vi "4-20mA Module (Main).vi"(7 "Name of Parent Panel":string="Main.vi", 9 "New Center Coords":T1={"Horizontal"=470, "Vertical"=200}, 10 "Config":variant, 11 "Main UI Message Queue":refnum<queue>) -> ()   [LabVIEW 2018, in "4-20mA Module.lvlib"]
doc: "This Continuous Measurement sample project is based on the Queued Message Handler template.\n\nThe Event Handling Loop generates messages based on user interface actions.\n\nThe Message Handling Loop processes messages generated by the Event Handling Loop, or by other messages. There are also Acquisition and Logging message handling loop subVIs, and a chart updating loop."
uses:
  4-20mA Module.lvlib
  support/Message Queue/Message Cluster.ctl
  <vilib>/Utility/miscctls.llb/LVPoint32TypeDef.ctl
  controls/UI Data.ctl
  controls/UI State.ctl
  Controls/4-20mA Module State Cluster.ctl
  Controls/4-20mA Module Config Cluster.ctl
  Controls/4-20mA Module Settings Cluster.ctl
  Pressure Transmitter/Pressure Transmitter Device Settings.ctl
  Pressure Reg Module/Pressure Regulator Device Settings.ctl
  Measure Instrument/State Enum.ctl
  Sequencing/Squence Update Cluster.ctl
  Controls/4-20mA Display Cluster.ctl
  Tag VIs/Tag FGV Operation Enum.ctl
  support/Message Queue/Enqueue Message (Single).vi
  support/User Event - Stop/User Event - Stop.lvlib
  support/Support Library.lvlib
  support/Message Queue/Message Queue.lvlib
  Measure Instrument/4-20mA Module Engine.lvlib
  Sequencing/Sequencing Library.lvlib
  Pressure Transmitter/Pressure Transmitter Library.lvlib
  Pressure Reg Module/Pressure Regulator Library.lvlib
  Shared Variables/Dynamic Shared Variables.lvlib
  Measure Instrument/Feed Module Engine.lvlib
  support/Command Log VIs/Command Logging.lvlib
  Settings Dialog.vi
  Report Generation/Report Generation.lvlib
panel:
  in  "Settings Dialog Button":bool
  out "User name":string
  out "Original Width 3":u32
  out "Original Width 2":u32
  out "Display Cluster":cluster{"Input":dbl, "Output":dbl} {"Output" format="%.2f"; "Input" format="%.2f"}
  out "Image Status":u16(ring)=2
  out "H/W":dbl
  out "Original Height":u32
  out "Original Width":u32
  out "Input Channel":string
  out "Log File path":path
  out "Status":string
  in  "Exit":bool
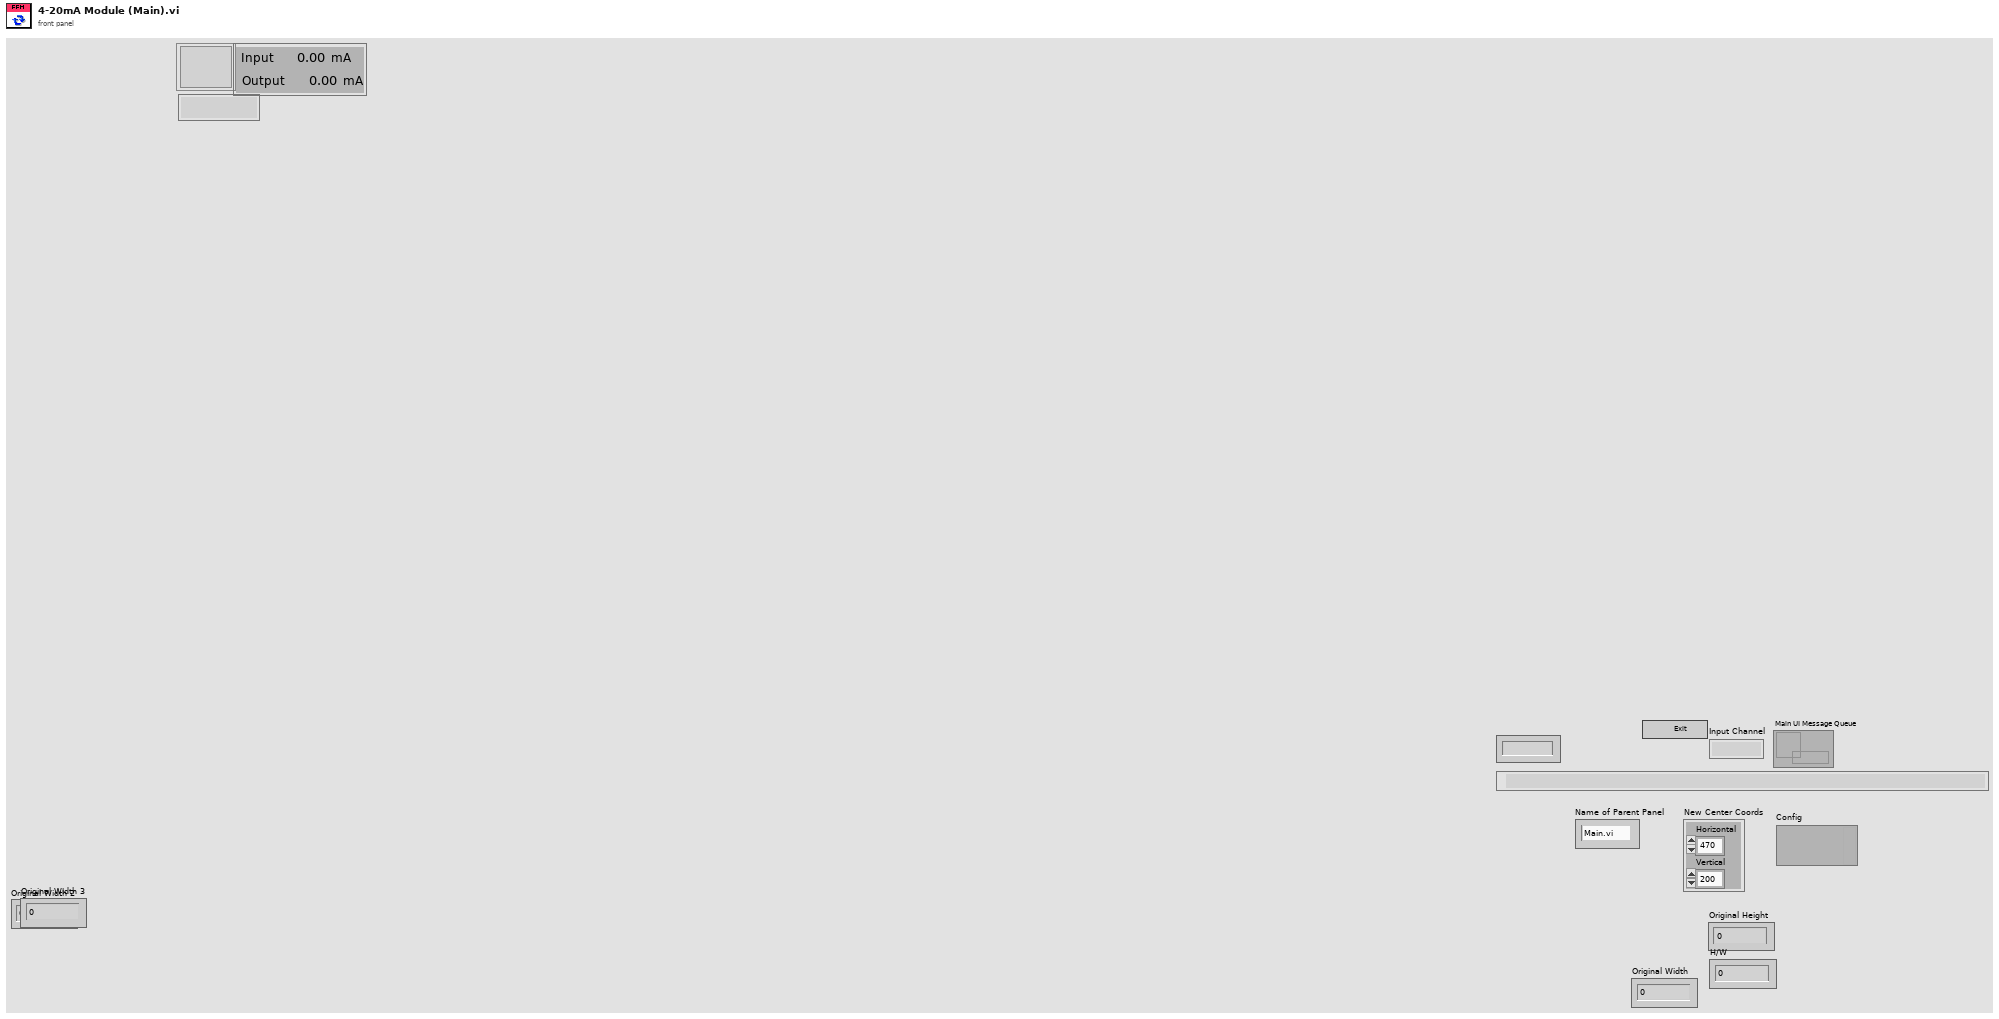
[diagram p1: front panel]
types:
  T1 = typedef "LVPoint32TypeDef.ctl" = cluster{"Horizontal":i32, "Vertical":i32}
  T2 = enum32{"Invalid", "Default", "Floating", "Floating/Auto-Hide", "Modal"}
  T3 = typedef "4-20mA Module.lvlib/4-20mA Module Config Cluster.ctl" = cluster{"GUID":string, "Drop Coords":T1, "Process Name":string, "User name":string, "Queue Name":string, "Settings":T4, "Settings Load Count":i32}
  T4 = typedef "4-20mA Module.lvlib/4-20mA Module Settings Cluster.ctl" = cluster{"Cycle Period":dbl, "PID 2 Parameters":cluster{"Input Device":enum16{"Default", "4-20mA"}, "Output Device":enum16{"Default", "Equilibar Pressure Reg", "Flow Regulator"}, "Setpoint":dbl, "PID gains":cluster{"proportional gain (Kc)":dbl, "integral time (Ti, min)":dbl, "derivative time (Td, min)":dbl}, "output range":cluster{"output low":dbl, "output high":dbl}}, "Manual Entry":dbl, "Auto?":bool, "4-20mA Input Settings":T5, "4-20mA Out Settings":T6, "Input Channel Tag Name ":string}
  T5 = typedef "Pressure Transmitter Library.lvlib/Pressure Transmitter Device Settings.ctl" = cluster{"Input Channel ":u16}
  T6 = typedef "Pressure Regulator Library.lvlib/Pressure Regulator Device Settings.ctl" = cluster{"Output DAQ Task":refnum<k21>}
  T7 = typedef "UI State.ctl" = enum16{"Idle", "Acquiring and Logging", "Waiting for Exit", "Waiting for Exit (Acq Stopped)", "Waiting for Exit (Log Stopped)", "Waiting for Stop", "Waiting for Stop (Acq Stopped)", "Waiting for Stop (Log Stopped)"}
  T8 = typedef "UI Data.ctl" = cluster{"Start Ref":refnum<vi>, "Trigger Ref":refnum<vi>, "Stop Ref":refnum<vi>, "Settings Ref":refnum<vi>, "Status Ref":refnum<vi>, "Exit Ref":refnum<vi>, "Data Ref":refnum<vi>}
  T9 = typedef "4-20mA Module.lvlib/4-20mA Module State Cluster.ctl" = cluster{"PRM Config":T3, "State":T10, "Start Time":timestamp, "Current Time":timestamp, "First Iteration":bool, "Data":cluster{"4-20mA Input":dbl, "PID 2 Process Variable":dbl, "PID 2 Output":dbl, "4-20mA Output":dbl}}
  T10 = typedef "Feed Module.lvlib/Feed Module Engine.lvlib/State Enum.ctl" = enum16{"Measuring", "Idle", "Paused"}
  T11 = typedef "LVPointTypeDef.ctl" = cluster{"Horizontal":i16, "Vertical":i16}
  T12 = typedef "4-20mA Module.lvlib/4-20mA Message Queues.ctl" = cluster{"UI":refnum<queue>, "Engine":refnum<queue>, "PR Display":refnum<queue>, "Setting Display":refnum<queue>}
  T13 = typedef "4-20mA Module.lvlib/4-20mA Display Cluster.ctl" = cluster{"Input 4-20":dbl, "Output 4-20":dbl, "Cycle Period":dbl, "Status":enum16{"Off", "On", "Not Initialized"}}
  T14 = typedef "Tag FGV Operation Enum.ctl" = enum16{"Init", "Set Notification Queue", "Create Tag", "Commit", "Write Tag (Numeric)", "Write Tag (Boolean)", "Read All Tags", "Read One Tag", "Delete Tag Category", "Set Alarm Parameters (Numeric)", "Set Alarm Parameters (Boolean)", "Enable All Alarms", "Disable All Alarms", "Delete All Tags", "Read Alarms", "Ack Alarm", "Read Alarm Parameters (Numeric)", "Read Alarm Parameters (Boolean)"}
  T15 = typedef "LVRectTypeDef.ctl" = cluster{"Left":i16, "Top":i16, "Right":i16, "Bottom":i16}
  T16 = cluster{"Shift":bool, "Ctrl":bool, "Alt":bool, "Cmd":bool, "Opt":bool}
  T17 = typedef "Sequencing Library.lvlib/Squence Update Cluster.ctl" = cluster{"Auto?":bool, "Manual Entry":dbl, "Setpoint":dbl}
  T18 = enum8{"Enabled", "Disabled", "Disabled and Grayed Out"}
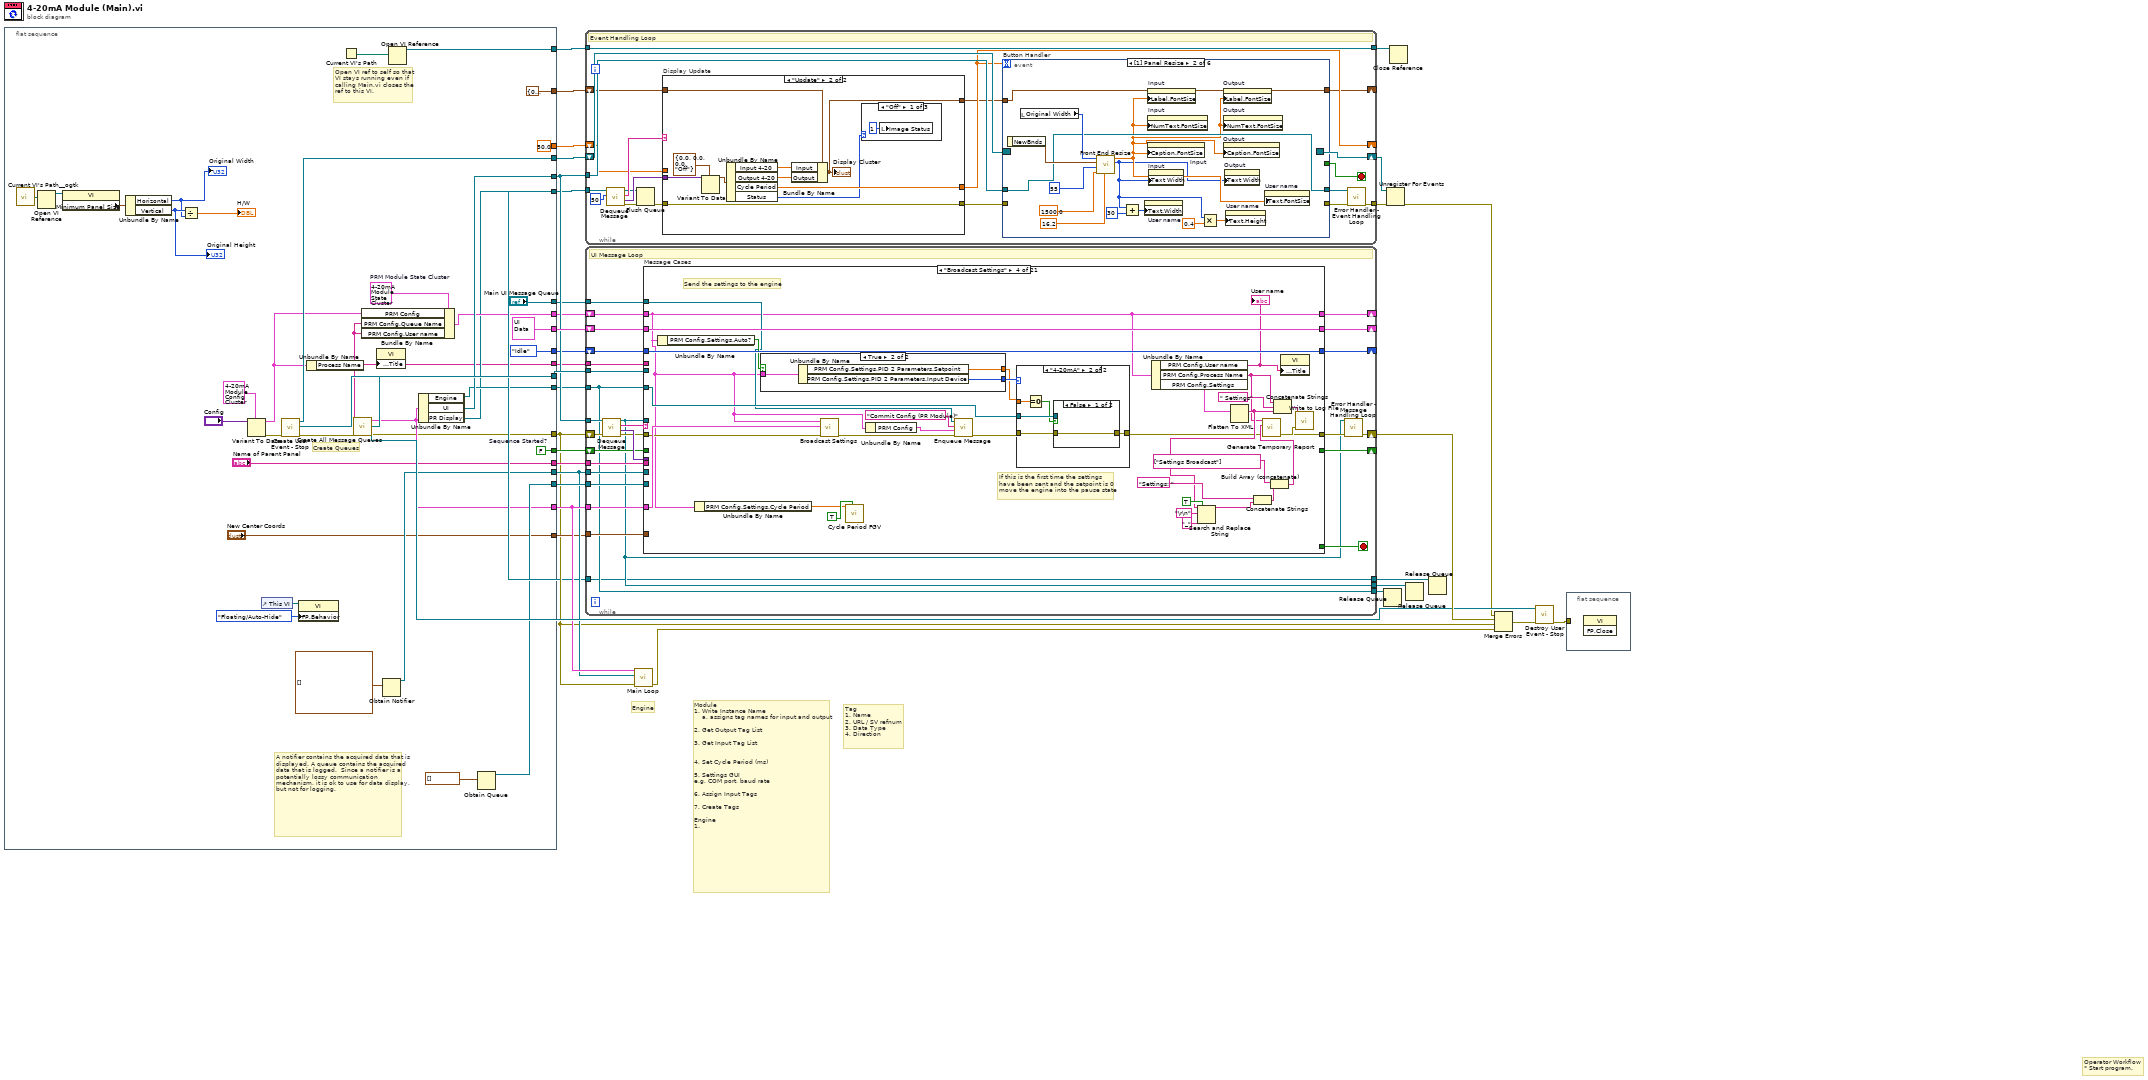
[diagram p0: block diagram]
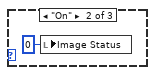
[diagram p3: hidden frame]
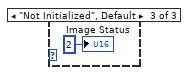
[diagram p4: hidden frame]
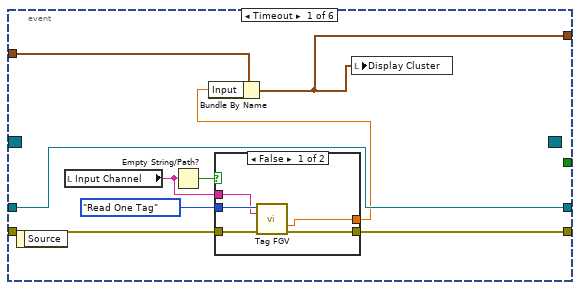
[diagram p5: hidden frame]
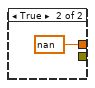
[diagram p6: hidden frame]
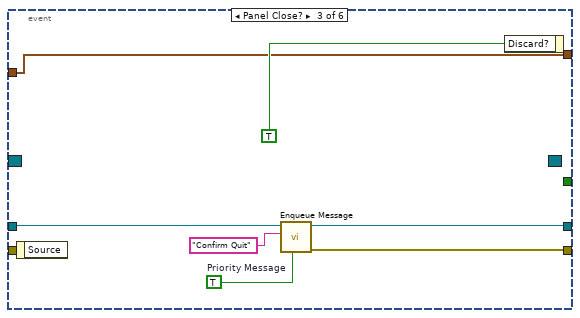
[diagram p7: hidden frame]
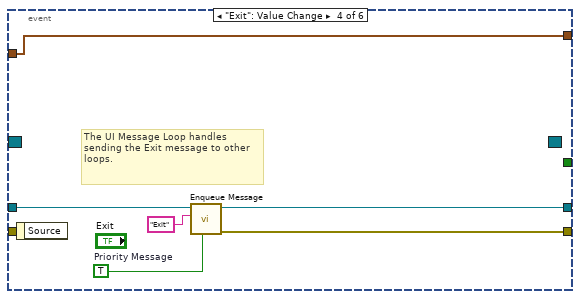
[diagram p8: hidden frame]
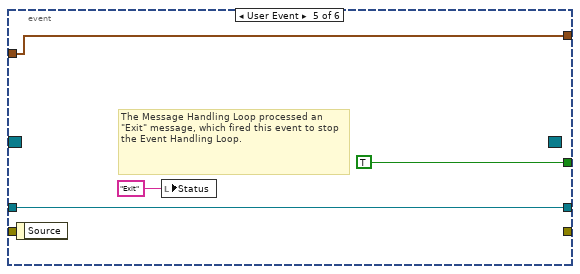
[diagram p9: hidden frame]
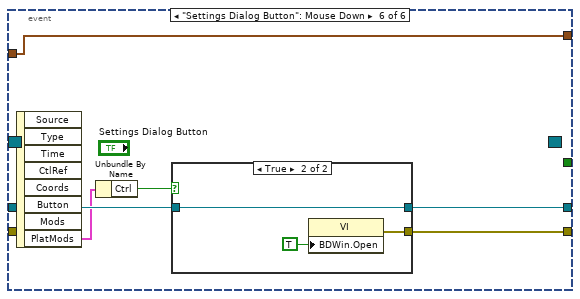
[diagram p10: hidden frame]
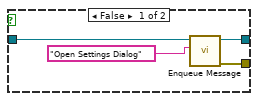
[diagram p11: hidden frame]
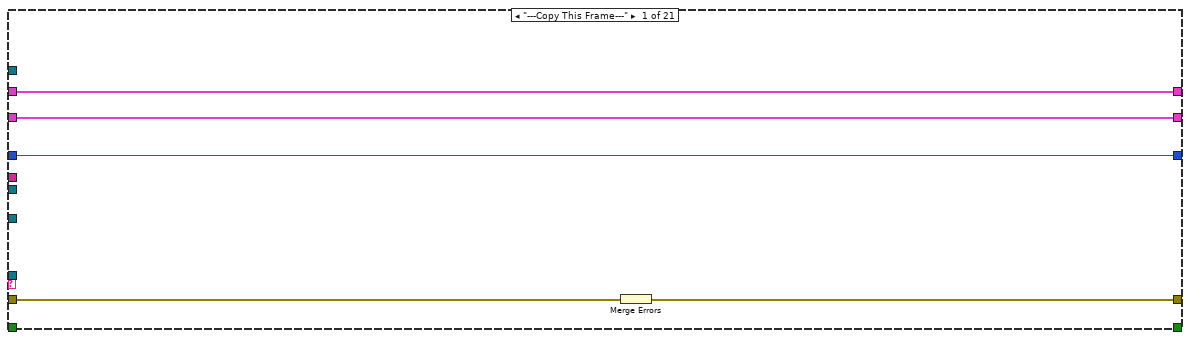
[diagram p12: hidden frame]
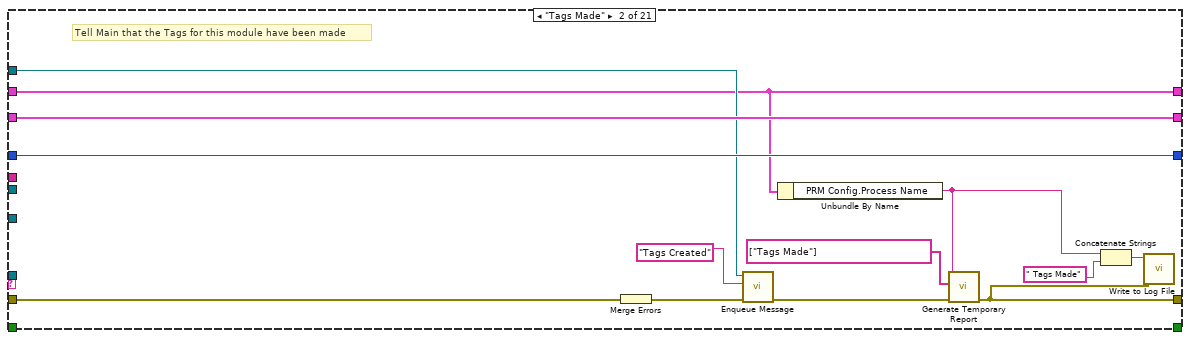
[diagram p13: hidden frame]
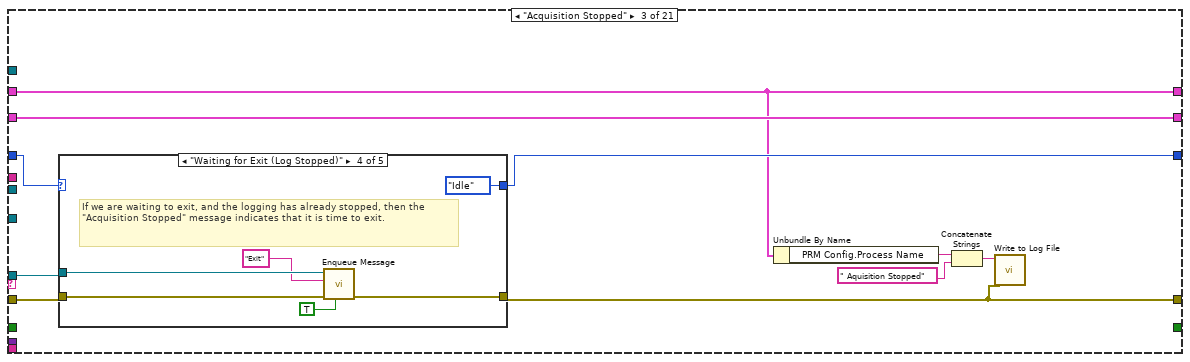
[diagram p14: hidden frame]
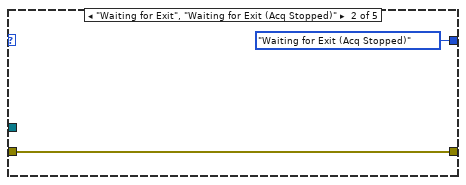
[diagram p16: hidden frame]
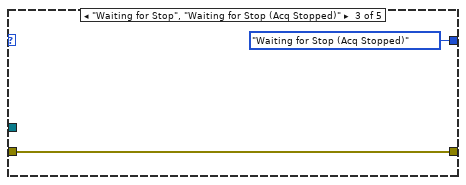
[diagram p17: hidden frame]
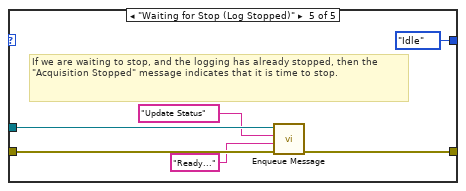
[diagram p18: hidden frame]
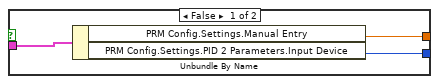
[diagram p19: hidden frame]
diagram:
  # "Engine"
  # "Operator Workflow\n* Start program."
  # "Module \n1. Write Instance Name\n    a. assigns tag names for input and output\n\n2. Get Output Tag List\n\n3. Get Input Tag List\n\n\n4. Set Cycle Period (ms)\n\n5. Settings GUI\ne.g. COM port, baud rate\n\n6. Assign Input Tags\n\n7. Create Tags\n\nEngine\n1."
  # "Tag\n1. Name\n2. URL / SV refnum\n3. Data Type\n4. Direction"
  n1 = flat-sequence {
    tunnel: [w68] -> w28
    tunnel: [w67] -> w27
    tunnel: [T8 {"Start Ref"=refnum, "Trigger Ref"=refnum, "Stop Ref"=refnum, "Settings Ref"=refnum, "Status Ref"=refnum, "Exit Ref"=refnum, "Data Ref"=refnum} ("Measurement UI Controls")] -> w24
    tunnel: [w64] -> w23
    tunnel: [UI_State."Idle" ("UI State")] -> w22
    tunnel: [w60] -> w21
    tunnel: [w59] -> w20
    tunnel: [w58] -> w18
    tunnel: [w57] -> w17
    tunnel: [w56] -> w15
    tunnel: ["Main UI Message Queue"] -> w14
    tunnel: ["Name of Parent Panel"] -> w13
    tunnel: ["New Center Coords"] -> w12
    tunnel: [w48] -> w10
    tunnel: [w47] -> w9
    tunnel: [w44] -> w8
    tunnel: [50.0 ("Cycle Period")] -> w7
    tunnel: [w42] -> w4
    tunnel: [w39] -> w2
    tunnel: [cluster{"Input":dbl, "Output":dbl} {"Input"=0.0, "Output"=0.0} ("Display Cluster 2")] -> w1
    frame #0 {
      w48 = FALSE  # Sequence Started?
      w51 = T9 {"PRM Config"={"GUID"="", "Drop Coords"={"Horizontal"=0, "Vertical"=0}, "Process Name"="", "User name"="", "Queue Name"="", "Settings"={"Cycle Period"=500.0, "PID 2 Parameters"={"Input Device"=enum."Default", "Output Device"=enum."Default", "Setpoint"=0.0, "PID gains"={"proportional gain (Kc)"=1.0, "integral time (Ti, min)"=0.01, "derivative time (Td, min)"=0.0}, "output range"={"output low"=0.0, "output high"=100.0}}, "Manual Entry"=0.0, "Auto?"=TRUE, "4-20mA Input Settings"={"Input Channel "=0}, "4-20mA Out Settings"={"Output DAQ Task"=""}, "Input Channel Tag Name "=""}, "Settings Load Count"=0}, "State"=enum."Idle", "Start Time"=timestamp(0 s since 1904-01-01), "Current Time"=timestamp(0 s since 1904-01-01), "First Iteration"=FALSE, "Data"={"4-20mA Input"=0.0, "PID 2 Process Variable"=0.0, "PID 2 Output"=0.0, "4-20mA Output"=0.0}}  # PRM Module State Cluster
      # "Create Queues"
      # "Open VI ref to self so that\nVI stays running even if\ncalling Main.vi closes the\nref to this VI."
      # "A notifier contains the acquired data that is displayed. A queue contains the acquired data that is logged.  Since a notifier is a potentially lossy communication mechanism, it is ok to use for data display, but not for logging."
      n2 = call <userlib>:"Current VI's Path__ogtk.vi"() -> ("Current VI's Path (+ Relative)"=w33:path)  [unwired: 1 in]
      n3 = Open VI Reference(vi path=w33) -> (vi reference=w34:refnum<vi>)  [unwired: 5 in, 1 out]
      n4 = property class="VI"(reference=w34) -> ("Minimum Panel Size"=w35:T11)  [unwired: 1 in, 2 out]
      n5 = Unbundle By Name(w35) -> ("Horizontal"=w36:i16, "Vertical"=w37:i16)
      "Original Width" <- w36
      "Original Height" <- w37
      n6 = Divide(x=w37, y=w36) -> (x/y=→"H/W":dbl)
      n7 = Variant To Data(type=T3 {"GUID"="", "Drop Coords"={"Horizontal"=0, "Vertical"=0}, "Process Name"="", "User name"="", "Queue Name"="", "Settings"={"Cycle Period"=500.0, "PID 2 Parameters"={"Input Device"=enum."Default", "Output Device"=enum."Default", "Setpoint"=0.0, "PID gains"={"proportional gain (Kc)"=1.0, "integral time (Ti, min)"=0.01, "derivative time (Td, min)"=0.0}, "output range"={"output low"=0.0, "output high"=100.0}}, "Manual Entry"=0.0, "Auto?"=TRUE, "4-20mA Input Settings"={"Input Channel "=0}, "4-20mA Out Settings"={"Output DAQ Task"=""}, "Input Channel Tag Name "=""}, "Settings Load Count"=0} ("Feed Module Config"), Variant="Config") -> (data=w53:T3, error out=w54:errorcluster)  [unwired: 1 in]
      n8 = control-ref of="This VI"() -> (w41:refnum<vi>)
      n9 = call "Create User Event - Stop.vi"("error in (no error)"=w54) -> ("error out"=w66:errorcluster, "User Event - Stop"=w67:refnum<user-event>, "Stop Event Registration Refnum"=w68:refnum<event-registration>)  [unwired: 8 in]
      n10 = property class="VI"(reference=w41, "FP.Behavior"=T2."Floating/Auto-Hide" ("Front Panel Window:Behavior")) -> ()  [unwired: 1 in, 2 out]
      n11 = Unbundle By Name(w53) -> ("Process Name"=w39:string)
      n12 = Current VI's Path() -> (path=w55:path)
      n13 = call "Create All Message Queues.vi"("error in (no error)"=w66, "Process Name"=w39) -> ("error out"=w47:errorcluster, "Message Queues"=w58:T12)  [unwired: 8 in]
      n14 = Bundle By Name(cluster=w51, "PRM Config"=w53, "PRM Config.Queue Name"=w39, "PRM Config.User name"=w39) -> (w44:T9)
      n15 = property class="VI"("Front Panel.Title"=w39) -> ()  [unwired: 2 in, 2 out]
      n16 = Obtain Notifier(notification data type=waveform(dbl)[] []) -> (notifier out=w57:refnum<notifier>)  [unwired: 3 in, 2 out]
      n17 = Open VI Reference(vi path=w55) -> (vi reference=w56:refnum<vi>)  [unwired: 5 in, 1 out]
      n18 = Unbundle By Name(w58) -> ("Engine"=w60:refnum<queue>, "UI"=w64:refnum<queue>, "PR Display"=w42:refnum<queue>)
      n19 = Obtain Queue(element data type=waveform(dbl)[] []) -> (queue out=w59:refnum<queue>)  [unwired: 4 in, 2 out]
    }
  }
  n20 = while {
    tunnel: w23 -> [w83]
    tunnel: [w85] -> w30
    shift-right: [w84] -> w25
    shift-left: w28 -> [w89]
    tunnel: [w82] -> w16
    tunnel: w15 -> [w82]
    tunnel: w4 -> [w81]
    shift-right: [w78] -> _
    shift-left: w7 -> [w77]
    shift-right: [w70] -> _
    shift-left: w1 -> [w69]
    stop <- w88 stop-if-true
    # "Event Handling Loop"
    n21 = call "Dequeue Message.vi"("timeout in ms (-1)"=50, "Message Queue"=w81) -> ("error out"=w74:errorcluster, "Message Data"=w79:variant, "Message"=w80:string, "dup Message Queue"=w75:refnum<queue>)  [unwired: 6 in]
    n22 = Flush Queue(queue=w75, error in (no error)=w74) -> (error out=w72:errorcluster)  [unwired: 2 out]
    n23 = case "Display Update" shown="\"Update\"" w80 {
      tunnel: w79 -> [_ w102]
      tunnel: [w92 w99] -> w78
      tunnel: w77 -> [w92 _]
      tunnel: [w91 w98] -> w73
      tunnel: w72 -> [w91 w98]
      tunnel: [w90 w94] -> w71
      tunnel: w69 -> [w90 w93]
      frame "False", Default {
      }
      frame "Update" {
        n24 = Variant To Data(type=T13 {"Input 4-20"=0.0, "Output 4-20"=0.0, "Cycle Period"=0.0, "Status"=enum."Off"} ("PRM Display Cluster"), Variant=w102) -> (data=w101:T13)  [unwired: 1 in, 1 out]
        n25 = Unbundle By Name(w101) -> ("Input 4-20"=w96:dbl, "Output 4-20"=w95:dbl, "Cycle Period"=w99:dbl, "Status"=w97:enum16{"Off", "On", "Not Initialized"})
        n26 = Bundle By Name(cluster=w93, "Input"=w96, "Output"=w95) -> (w94:cluster{"Input":dbl, "Output":dbl})
        "Display Cluster" <- w94
        n27 = case shown="\"Off\"" w97 {
          frame "Off" {
            n28 = local write "Image Status"(u16 1 ("Ring")) -> ()
          }
          frame "On" {
            n29 = local write "Image Status"(u16 0 ("Ring")) -> ()
          }
          frame "Not Initialized", Default {
            "Image Status" <- u16 2 ("Ring")
          }
        }
      }
    }
    n30 = event "Button Handler" shown="[1] Panel Resize" {
      selector: w89 -> [_ _ _ _ _ _]
      dyn-events: [_ _ _ _ _ _] -> w84
      timeout: w78 -> [_ _ _ _ _ _]
      tunnel: [_ _ _ _ TRUE ("Discard?") _] -> w88
      tunnel: w83 -> [w114 w127 w137 w143 w148 w154]
      tunnel: [w109 _ w135 w146 _ w156] -> w86
      tunnel: [w114 w127 w136 w142 w148 w155] -> w87
      tunnel: w73 -> [w110 _ _ _ _ _]
      tunnel: w71 -> [w107 w133 w134 w141 w147 w151]
      tunnel: [w106 w133 w134 w141 w147 w151] -> w70
      event Timeout {
        n31 = event-data() -> ()  [unwired: 1 in, 1 out]
        n32 = local read "Input Channel"() -> (w111:string)
        n33 = Empty String/Path?(string/path=w111) -> (empty?=w113:bool)
        n34 = case shown="False" w113 {
          tunnel: Tag_FGV_Operation_Enum."Read One Tag" ("Operation") -> [w119 _]
          tunnel: [w118 nan ("Tag Value")] -> w108
          tunnel: [w117 _] -> w109
          tunnel: w111 -> [w116 _]
          tunnel: w110 -> [w115 _]
          frame False {
            n35 = call "Tag FGV.vi"("Operation"=w119, "Tag Name"=w116, "error in (no error)"=w115) -> ("Tag Value"=w118:dbl, "error out"=w117:errorcluster)  [unwired: 5 in, 6 out]
          }
          frame True {
          }
        }
        n36 = Bundle By Name(cluster=w107, "Input"=w108) -> (w106:cluster{"Input":dbl, "Output":dbl})
        n37 = local write "Display Cluster"(w106) -> ()
      }
      event Panel Resize {
        n38 = event-data() -> ("NewBnds"=w132:T15)  [unwired: 1 in]
        n39 = local read "Original Width"() -> (w131:u32)
        n40 = call "Front End Resize.vi"("Starting Font"=16.2, "Area to Font Division"=1500.0, "Original Text Box Width"=55, "NewBnds"=w132, "Original Panel Width"=w131) -> ("New Text Box Width"=w122:u64, "New Font Size"=w126:dbl)  [unwired: 5 in]
        n41 = Add(x=w122, y=u64 30) -> (x+y=w124:u64)
        n42 = property on="User name" class="Str"("Text.Width"=w124) -> ()  [unwired: 2 in, 2 out]
        n43 = property on="Input" class="DigNum (strict)"("Label.FontSize"=w126) -> ()  [unwired: 2 in, 2 out]
        n44 = property on="Input" class="DigNum (strict)"("NumText.FontSize"=w126) -> ()  [unwired: 2 in, 2 out]
        n45 = property on="Input" class="DigNum (strict)"("Caption.FontSize"=w126) -> ()  [unwired: 2 in, 2 out]
        n46 = property on="Input" class="DigNum (strict)"("Text Width"=w122) -> ()  [unwired: 2 in, 2 out]
        n47 = Multiply(x=w122, y=0.4) -> (x*y=w121:dbl)
        n48 = property on="Output" class="DigNum (strict)"("Label.FontSize"=w126) -> ()  [unwired: 2 in, 2 out]
        n49 = property on="Output" class="DigNum (strict)"("NumText.FontSize"=w126) -> ()  [unwired: 2 in, 2 out]
        n50 = property on="Output" class="DigNum (strict)"("Caption.FontSize"=w126) -> ()  [unwired: 2 in, 2 out]
        n51 = property on="Output" class="DigNum (strict)"("Text Width"=w122) -> ()  [unwired: 2 in, 2 out]
        n52 = property on="User name" class="Str"("Text.Height"=w121) -> ()  [unwired: 2 in, 2 out]
        n53 = property on="User name" class="Str"("Text.FontSize"=w126) -> ()  [unwired: 2 in, 2 out]
      }
      event Panel Close? {
        w138 = TRUE  # Priority Message
        n54 = event-data() -> ()  [unwired: 1 in, 1 out]
        n55 = call-poly "Enqueue Message.vi"("Priority Message? (F)"=w138, "Message"="Confirm Quit", "Message Queue"=w137) -> ("error out"=w135:errorcluster, "dup Message Queue"=w136:refnum<queue>)  [unwired: 7 in]
        n56 = event-data("Discard?"=TRUE) -> ()  [unwired: 1 in, 1 out]
      }
      event "Exit": Value Change {
        w144 = TRUE  # Priority Message
        # "The UI Message Loop handles sending the Exit message to other loops."
        n57 = event-data() -> ()  [unwired: 1 in, 1 out]
        n58 = call-poly "Enqueue Message.vi"("Priority Message? (F)"=w144, "Message"="Exit", "Message Queue"=w143) -> ("error out"=w146:errorcluster, "dup Message Queue"=w142:refnum<queue>)  [unwired: 7 in]
      }
      event User Event {
        # "The Message Handling Loop processed an \"Exit\" message, which fired this event to stop the Event Handling Loop."
        n59 = event-data() -> ()  [unwired: 1 in, 1 out]
        n60 = local write "Status"("Exit" ("Exit String")) -> ()
      }
      event "Settings Dialog Button": Mouse Down {
        n61 = event-data() -> ("PlatMods"=w153:T16)  [unwired: 1 in, 7 out]
        n62 = Unbundle By Name(w153) -> ("Ctrl"=w152:bool)
        n63 = case shown="True" w152 {
          tunnel: [w160 w161] -> w156
          tunnel: [w159 w162] -> w155
          tunnel: w154 -> [w158 w162]
          frame False {
            n64 = call-poly "Enqueue Message.vi"("Message"="Open Settings Dialog", "Message Queue"=w158) -> ("error out"=w160:errorcluster, "dup Message Queue"=w159:refnum<queue>)  [unwired: 8 in]
          }
          frame True {
            n65 = property class="VI"("BDWin.Open"=TRUE ("Block Diagram Window:Open")) -> (error out=w161:errorcluster)  [unwired: 2 in, 1 out]
          }
        }
      }
    }
    n66 = call "Error Handler - Event Handling Loop.vi"("error in (no error)"=w86, "Message Queue"=w87) -> ("dup error in"=w85:errorcluster)  [unwired: 8 in, 1 out]
  }
  n67 = while {
    tunnel: w23 -> [w185]
    tunnel: w27 -> [w189]
    shift-right: [w180] -> w31
    shift-left: w9 -> [w188]
    shift-right: [w183] -> _
    shift-left: w24 -> [w184]
    tunnel: w17 -> [w172]
    tunnel: w20 -> [w182]
    shift-right: [w179] -> _
    shift-left: w22 -> [w174]
    tunnel: w21 -> [w166]
    tunnel: w18 -> [w171]
    tunnel: w14 -> [w175]
    tunnel: w13 -> [w178]
    tunnel: w2 -> [w177]
    tunnel: w12 -> [w176]
    shift-right: [w169] -> _
    shift-left: w10 -> [w170]
    shift-right: [w167] -> _
    shift-left: w8 -> [w168]
    tunnel: [w166] -> w6
    tunnel: [w165] -> w5
    tunnel: [w164] -> w3
    tunnel: w4 -> [w164]
    stop <- w190 stop-if-true
    # "UI Message Loop"
    n68 = call "Dequeue Message.vi"("error in (no error)"=w188, "Message Queue"=w185) -> ("error out"=w173:errorcluster, "Message Data"=w186:variant, "Message"=w187:string, "dup Message Queue"=w165:refnum<queue>)  [unwired: 6 in]
    n69 = case "Message Cases" shown="\"Broadcast Settings\"" w187 {
      selector: w187 -> [_ _ _ _ _ _ _ _ _ _ _ _ _ _ _ _ _ _ _ _ w651]
      tunnel: w165 -> [_ _ w214 _ w293 _ w351 w367 w399 w427 _ w467 w483 w499 w532 w550 _ _ w626 _ _]
      tunnel: w173 -> [w195 w208 w215 w263 w292 w319 w336 w366 w402 w430 w452 w462 _ w500 w525 w548 w576 w588 w611 w639 _]
      tunnel: [w194 w196 w210 w238 w287 w320 w325 w355 w390 w404 w452 w454 w476 w495 w531 w541 w573 w596 w604 w640 w646] -> w181
      tunnel: [_ _ _ _ _ _ _ _ _ TRUE _ _ _ _ _ _ _ _ _ _ _] -> w190
      tunnel: w186 -> [_ _ _ _ _ w322 _ _ w401 w416 _ _ w482 _ _ _ _ _ _ w638 _]
      tunnel: w189 -> [_ _ _ _ _ _ _ _ _ w429 _ _ _ _ _ _ _ _ _ _ _]
      tunnel: w184 -> [w193 w207 w218 w268 w295 w324 w348 w364 w403 w428 w451 w463 w485 w503 w533 w564 w582 w595 w623 w635 w654]
      tunnel: [w193 w207 w218 w268 w295 w324 w348 w364 w403 w428 w450 w463 w485 w503 w533 w564 w582 w595 w623 w635 w654] -> w183
      tunnel: w182 -> [_ _ _ _ _ _ _ _ _ w422 _ _ _ _ _ _ _ _ _ _ _]
      tunnel: w174 -> [w192 w206 w217 w267 w294 w318 w337 _ w394 _ _ _ w484 w502 w528 _ _ _ w612 w630 w653]
      tunnel: [w192 w206 w216 w267 w291 w318 w338 UI_State."Acquiring and Logging" ("UI State") w394 UI_State."Idle" ("UI State") UI_State."Idle" ("UI State") UI_State."Idle" ("UI State") w484 w501 w528 UI_State."Acquiring and Logging" ("UI State") UI_State."Acquiring and Logging" ("UI State") UI_State."Acquiring and Logging" ("UI State") w613 w630 w653] -> w179
      tunnel: w166 -> [_ _ _ w262 _ _ w335 _ _ w420 _ _ _ _ _ _ w580 w593 w610 _ _]
      tunnel: w178 -> [_ _ _ _ _ _ _ _ _ _ _ w461 _ _ _ _ _ _ _ _ _]
      tunnel: w177 -> [_ _ _ _ _ _ _ _ _ _ _ w458 _ _ _ _ _ _ _ _ _]
      tunnel: w176 -> [_ _ _ _ _ _ _ _ _ _ _ w460 _ _ _ _ _ _ _ _ _]
      tunnel: w175 -> [_ w204 _ w255 _ _ _ _ _ w414 _ _ _ _ _ _ _ _ _ _ _]
      tunnel: w172 -> [_ _ _ _ _ _ _ _ _ w426 _ _ _ _ _ _ _ _ _ _ _]
      tunnel: w171 -> [_ _ _ w266 _ _ _ _ _ _ _ _ _ _ w526 _ _ _ _ _ _]
      tunnel: w168 -> [w191 w200 w209 w250 w286 w317 w329 w354 w389 w411 w443 w453 w475 w494 w529 w543 w578 w590 w603 w629 w652]
      tunnel: w170 -> [_ _ _ _ _ _ _ w363 _ _ _ _ _ _ _ _ _ _ _ _ _]
      tunnel: [_ _ _ _ _ _ _ w360 _ _ _ _ _ _ _ _ _ _ _ _ _] -> w169
      tunnel: [w191 w200 w209 w250 w286 w317 w329 w354 w389 w411 w443 w453 w474 w494 w523 w543 w578 w590 w603 w629 w652] -> w167
      frame "---Copy This Frame---" {
        # "Duplicate this frame when creating new messages.  Change this comment in the duplicated frame to describe this message."
        n70 = Merge Errors(w195) -> (w194:errorcluster)
      }
      frame "Tags Made" {
        # "Tell Main that the Tags for this module have been made"
        # "Duplicate this frame when creating new messages.  Change this comment in the duplicated frame to describe this message."
        n71 = Merge Errors(w208) -> (w203:errorcluster)
        n72 = call-poly "Enqueue Message.vi"("error in (no error)"=w203, "Message"="Tags Created", "Message Queue"=w204) -> ("error out"=w197:errorcluster)  [unwired: 7 in, 1 out]
        n73 = Unbundle By Name(w200) -> ("PRM Config.Process Name"=w198:string)
        n74 = call "Generate Temporary Report.vi"("error in (no error)"=w197, "Line of Events"=string[] ["Tags Made"], "Module Name"=w198) -> ("error out"=w196:errorcluster)  [unwired: 8 in]
        n75 = Concatenate Strings(w198, " Tags Made" ("text")) -> (w201:string)
        n76 = call "Write to Log File.vi"("error in"=w196, "text"=w201) -> ()  [unwired: 9 in, 1 out]
      }
      frame "Acquisition Stopped" {
        # "Logic for determining what action to take when the acquisition has stopped."
        n77 = case shown="\"Waiting for Exit (Log Stopped)\"" w217 {
          selector: w217 -> [w220 _ _ _ _]
          tunnel: [w220 UI_State."Waiting for Exit (Acq Stopped)" ("UI State") UI_State."Waiting for Stop (Acq Stopped)" ("UI State") UI_State."Idle" ("UI State") UI_State."Idle" ("UI State")] -> w216
          tunnel: w215 -> [w219 w221 w223 w229 w235]
          tunnel: [w219 w221 w223 w228 w234] -> w210
          tunnel: w214 -> [_ _ _ w227 w233]
          frame Default {
          }
          frame "Waiting for Exit", "Waiting for Exit (Acq Stopped)" {
          }
          frame "Waiting for Stop", "Waiting for Stop (Acq Stopped)" {
          }
          frame "Waiting for Exit (Log Stopped)" {
            # "If we are waiting to exit, and the logging has already stopped, then the \"Acquisition Stopped\" message indicates that it is time to exit."
            n78 = call-poly "Enqueue Message.vi"("Priority Message? (F)"=TRUE, "error in (no error)"=w229, "Message"="Exit", "Message Queue"=w227) -> ("error out"=w228:errorcluster)  [unwired: 6 in, 1 out]
          }
          frame "Waiting for Stop (Log Stopped)" {
            # "If we are waiting to stop, and the logging has already stopped, then the \"Acquisition Stopped\" message indicates that it is time to stop."
            n79 = call-poly "Enqueue Message.vi"("error in (no error)"=w235, "Message Data"="Ready..." ("Message"), "Message"="Update Status", "Message Queue"=w233) -> ("error out"=w234:errorcluster)  [unwired: 6 in, 1 out]
          }
        }
        n80 = Unbundle By Name(w209) -> ("PRM Config.Process Name"=w213:string)
        n81 = Concatenate Strings(w213, " Aquisition Stopped" ("text")) -> (w211:string)
        n82 = call "Write to Log File.vi"("error in"=w210, "text"=w211) -> ()  [unwired: 9 in, 1 out]
      }
      frame "Broadcast Settings" {
        # "If this is the first time the settings\nhave been sent and the setpoint is 0 \nmove the engine into the pause state"
        # "Send the settings to the engine"
        # "Send the 'Update Settings' message to the Logging and Acquisition message loops."
        n83 = Unbundle By Name(w250) -> ("PRM Config.Settings.Auto?"=w259:bool)
        n84 = Unbundle By Name(w250) -> ("PRM Config.Settings.Cycle Period"=w264:dbl)
        n85 = case shown="True" w259 {
          tunnel: [w269 w274] -> w261
          tunnel: [w270 w273] -> w260
          tunnel: w250 -> [w271 w272]
          frame False {
            n86 = Unbundle By Name(w271) -> ("PRM Config.Settings.Manual Entry"=w270:dbl, "PRM Config.Settings.PID 2 Parameters.Input Device"=w269:enum16{"Default", "4-20mA"})
          }
          frame True {
            n87 = Unbundle By Name(w272) -> ("PRM Config.Settings.PID 2 Parameters.Setpoint"=w273:dbl, "PRM Config.Settings.PID 2 Parameters.Input Device"=w274:enum16{"Default", "4-20mA"})
          }
        }
        n88 = call "Broadcast Settings.vi"("error in (no error)"=w263, "Message Queues"=w266, "PRM Module State Cluster"=w250) -> ("error out"=w257:errorcluster)  [unwired: 8 in]
        n89 = call "Cycle Period FGV.vi"("Write"=TRUE, "Cycle Period In (ms)"=w264) -> ()  [unwired: 8 in, 2 out]
        n90 = Unbundle By Name(w250) -> ("PRM Config"=w254:T3)
        n91 = call-poly "Enqueue Message.vi"("error in (no error)"=w257, "Message Data"=w254, "Message"="Commit Config (PR Module)", "Message Queue"=w255) -> ("error out"=w256:errorcluster)  [unwired: 6 in, 1 out]
        n92 = case shown="\"4-20mA\"" w261 {
          tunnel: w256 -> [w275 w280]
          tunnel: w262 -> [_ w279]
          tunnel: [w275 w278] -> w239
          tunnel: w260 -> [_ w277]
          frame "Default", Default {
          }
          frame "4-20mA" {
            n93 = Equal To 0?(x=w277) -> (x = 0?=w276:bool)
            n94 = case shown="False" w276 {
              tunnel: w280 -> [w281 w285]
              tunnel: w279 -> [_ w284]
              tunnel: [w281 w283] -> w278
              frame False {
              }
              frame True {
                n95 = call-poly "Enqueue Message.vi"("error in (no error)"=w285, "Message"="Pause", "Message Queue"=w284) -> ("error out"=w283:errorcluster)  [unwired: 7 in, 1 out]
              }
            }
          }
        }
        n96 = Unbundle By Name(w250) -> ("PRM Config.User name"=w237:string, "PRM Config.Process Name"=w240:string, "PRM Config.Settings"=w251:T4)
        "User name" <- w237
        n97 = Flatten To XML(anything=w251) -> (xml string=w241:string)
        n98 = Search and Replace String(replace all?=TRUE ("replace all? (F)"), input string=w241, search string="\r\n", replace string="_" ("replace string (\"\")")) -> (result string=w245:string)  [unwired: 4 in, 3 out]
        n99 = Concatenate Strings("Settings: " ("string"), w245) -> (w247:string)
        n100 = Build Array (concatenate)(string[] ["Settings Broadcast"] ("Line of Events"), w247) -> (w249:string[])
        n101 = call "Generate Temporary Report.vi"("error in (no error)"=w239, "Line of Events"=w249, "Module Name"=w240) -> ("error out"=w238:errorcluster)  [unwired: 8 in]
        n102 = Concatenate Strings(w240, " Settings" ("text"), w241) -> (w252:string)
        n103 = property class="VI"("Front Panel.Title"=w237) -> ()  [unwired: 2 in, 2 out]
        n104 = call "Write to Log File.vi"("error in"=w239, "text"=w252) -> ()  [unwired: 9 in, 1 out]
      }
      frame "Confirm Quit" {
        # "Confirm Quit - Message that can confirm whether or not the user wants to exit the application."
        n105 = case shown="\"Acquiring and Logging\"" w294 {
          tunnel: w293 -> [w300 w306]
          tunnel: w292 -> [w299 w304]
          tunnel: [w296 w303] -> w287
          tunnel: [UI_State."Idle" ("UI State") w302] -> w291
          frame Default {
            # "If 'Confirm Quit' comes in while the system is idle, there is no need for a confirmation message."
            n106 = call-poly "Enqueue Message.vi"("Priority Message? (F)"=TRUE, "error in (no error)"=w299, "Message"="Exit", "Message Queue"=w300) -> ("error out"=w296:errorcluster)  [unwired: 6 in, 1 out]
          }
          frame "Acquiring and Logging" {
            n107 = Two Button Dialog(message="Are you sure you want to quit while the acquisition is running?" ("Confirm Quit Message"), 1:"No" ("No"), 2:"Yes" ("Yes")) -> (T button?=w305:bool)
            n108 = case shown="True" w305 {
              tunnel: w306 -> [_ w316]
              tunnel: w304 -> [w310 w315]
              tunnel: [w310 w314] -> w303
              tunnel: [UI_State."Acquiring and Logging" ("UI State") UI_State."Waiting for Exit" ("UI State")] -> w302
              frame False {
                # "User did not want to quit."
              }
              frame True {
                n109 = call-poly "Enqueue Message.vi"("error in (no error)"=w315, "Message"="Stop", "Message Queue"=w316) -> ("error out"=w314:errorcluster)  [unwired: 7 in, 1 out]
              }
            }
          }
        }
        n110 = Unbundle By Name(w286) -> ("PRM Config.Process Name"=w290:string)
        n111 = Concatenate Strings(w290, " Confirm Quit" ("text")) -> (w288:string)
        n112 = call "Write to Log File.vi"("error in"=w287, "text"=w288) -> ()  [unwired: 9 in, 1 out]
      }
      frame "Display Log File Path" {
        n113 = Variant To Data(error in=w319, type=path "", Variant=w322) -> (data=→"Log File path":path, error out=w320:errorcluster)
      }
      frame "E-Stop" {
        # "E-Stop pauses the engine"
        # "Message Acquisition and Logging loops to stop"
        # "Enable: Start, Exit, Settings\nDisable: Stop"
        # "Stop the pumps."
        n114 = Unbundle By Name(w348) -> ("Trigger Ref"=w339:refnum<vi>, "Stop Ref"=w340:refnum<vi>, "Start Ref"=w343:refnum<vi>, "Exit Ref"=w342:refnum<vi>, "Settings Ref"=w341:refnum<vi>)
        n115 = call-poly "Enqueue Message.vi"("error in (no error)"=w336, "Message Data"="Ready..." ("Ready..."), "Message"="Update Status", "Message Queue"=w351) -> ("error out"=w333:errorcluster)  [unwired: 6 in, 1 out]
        n116 = Build Array(w343, w342, w341) -> (w346:refnum<vi>[])
        n117 = Build Array(w339, w340) -> (w345:refnum<vi>[])
        n118 = call-poly "Enqueue Message.vi"("error in (no error)"=w333, "Message"="Pause", "Message Queue"=w335) -> ("error out"=w332:errorcluster)  [unwired: 7 in, 1 out]
        n119 = call "Set Enable State on Multiple Controls.vi"("Enable?"=FALSE, "Controls"=w345) -> ()  [unwired: 10 in]
        n120 = call "Set Enable State on Multiple Controls.vi"("Enable?"=TRUE, "Controls"=w346) -> ()  [unwired: 10 in]
        n121 = case shown="\"Waiting for Exit\"" w337 {
          selector: w337 -> [_ w353]
          tunnel: [UI_State."Waiting for Stop" ("UI State") w353] -> w338
          frame Default {
          }
          frame "Waiting for Exit" {
          }
        }
        n122 = Merge Errors(w332) -> (w326:errorcluster)
        n123 = Unbundle By Name(w329) -> ("PRM Config.Process Name"=w327:string)
        n124 = call "Generate Temporary Report.vi"("error in (no error)"=w326, "Line of Events"=string[] ["E-STOP"], "Module Name"=w327) -> ("error out"=w325:errorcluster)  [unwired: 8 in]
        n125 = Concatenate Strings(w327, " E-STOP" ("text")) -> (w330:string)
        n126 = call "Write to Log File.vi"("error in"=w325, "text"=w330) -> ()  [unwired: 9 in, 1 out]
      }
      frame "Sequence Start" {
        # "Clear chart"
        # "Message Acquisition and Logging loops to start"
        # "Enable: Stop\nDisable: Start, Exit, Settings"
        # "Stop the pumps."
        n127 = Unbundle By Name(w364) -> ("Trigger Ref"=w371:refnum<vi>, "Stop Ref"=w372:refnum<vi>, "Start Ref"=w375:refnum<vi>, "Exit Ref"=w374:refnum<vi>, "Settings Ref"=w373:refnum<vi>, "Data Ref"=w369:refnum<vi>)
        n128 = property class="WFChart (strict)"(reference=w369, "History Data"=waveform(dbl)[][] []) -> ()  [unwired: 1 in, 2 out]
        n129 = Build Array(w375, w374, w373) -> (w378:refnum<vi>[])
        n130 = Build Array(w371, w372) -> (w377:refnum<vi>[])
        n131 = call-poly "Enqueue Message.vi"("error in (no error)"=w366, "Message"="Broadcast settings", "Message Queue"=w367) -> ("error out"=w361:errorcluster, "dup Message Queue"=w362:refnum<queue>)  [unwired: 7 in]
        n132 = call "Set Enable State on Multiple Controls.vi"("Enable?"=TRUE, "Controls"=w377) -> ()  [unwired: 10 in]
        n133 = call "Set Enable State on Multiple Controls.vi"("Enable?"=FALSE, "Controls"=w378) -> ()  [unwired: 10 in]
        n134 = case shown="False" w363 {
          selector: w363 -> [_ w385]
          tunnel: [w384 w385] -> w360
          tunnel: w361 -> [w383 w386]
          tunnel: w362 -> [w381 _]
          tunnel: [w380 w386] -> w359
          frame False {
            w384 = TRUE  # Sequence Started?
            n135 = call-poly "Enqueue Message.vi"("error in (no error)"=w383, "Message"="Start Loops", "Message Queue"=w381) -> ("error out"=w380:errorcluster)  [unwired: 7 in, 1 out]
          }
          frame True {
          }
        }
        n136 = Merge Errors(w359) -> (w355:errorcluster)
        n137 = Unbundle By Name(w354) -> ("PRM Config.Process Name"=w358:string)
        n138 = Concatenate Strings(w358, " Sequence Start" ("text")) -> (w356:string)
        n139 = call "Write to Log File.vi"("error in"=w355, "text"=w356) -> ()  [unwired: 9 in, 1 out]
      }
      frame "Error" {
        # "Stop if there is an error"
        # "Error - Check the error message data and respond accordingly. This message is sent by the \"Error Handler\" VIs at the end of each loop in this application."
        n140 = Variant To Data(error in=w402, type=errorcluster {"status"=FALSE, "code"=0, "source"=""} ("error out"), Variant=w401) -> (data=w387:errorcluster, error out=w396:errorcluster)
        n141 = call <vilib>:"Simple Error Handler.vi"("error in (no error)"=w387) -> ()  [unwired: 4 in, 5 out]
        n142 = call-poly "Enqueue Message.vi"("Priority Message? (F)"=TRUE, "Message"="Exit", "Message Queue"=w399) -> ("error out"=w395:errorcluster)  [unwired: 7 in, 1 out]
        n143 = Merge Errors(w395, w396) -> (w390:errorcluster)
        n144 = call <vilib>:"General Error Handler.vi"("error in (no error)"=w387) -> ("message"=w388:string)  [unwired: 10 in, 4 out]
        n145 = Unbundle By Name(w389) -> ("PRM Config.Process Name"=w393:string)
        n146 = Concatenate Strings(w393, " Error: " ("text"), w388) -> (w391:string)
        n147 = call "Write to Log File.vi"("error in"=w390, "text"=w391) -> ()  [unwired: 9 in, 1 out]
      }
      frame "Exit" {
        w418 = TRUE  # Delete Module?
        # "Don't check the error outs. The acquisition and logging queues may have already been released."
        # "Close references owned by the Main VI."
        # "Stop the VI"
        # "Exit - Fire the User Event to stop the Event Handling Loop.  Also send Exit messages to the Acquisition and Logging loops."
        n148 = Release Queue(queue=w427, error in (no error)=w430) -> (error out=w425:errorcluster)  [unwired: 1 in, 2 out]
        n149 = call "Fire User Event - Stop.vi"("User Event - Stop"=w429) -> ("error out"=w409:errorcluster)  [unwired: 10 in]
        n150 = Release Notifier(notifier=w426, error in (no error)=w425) -> (error out=w424:errorcluster)  [unwired: 1 in, 2 out]
        n151 = Variant To Data(type=w418, Variant=w416) -> (data=w417:bool, error out=w419:errorcluster)  [unwired: 1 in]
        n152 = flat-sequence {
          tunnel: w420 -> [w436]
          tunnel: [w432] -> w410
          tunnel: w409 -> [w432]
          tunnel: [w437] -> w408
          tunnel: w410 -> [w437]
          frame #0 {
            n153 = call-poly "Enqueue Message.vi"("Message"="Stop", "Message Queue"=w436) -> ("dup Message Queue"=w434:refnum<queue>)  [unwired: 8 in, 1 out]
            n154 = call-poly "Enqueue Message.vi"("Message"="Exit", "Message Queue"=w434) -> ()  [unwired: 8 in, 2 out]
          }
          frame #1 {
            n155 = Wait (ms)(milliseconds to wait=u32 1000) -> ()  [unwired: 1 out]
          }
        }
        n156 = Release Queue(queue=w422, error in (no error)=w424) -> (error out=w423:errorcluster)  [unwired: 1 in, 2 out]
        n157 = Select(t=w418, s=w419, f=w417) -> (s? t:f=w415:bool)
        n158 = case "Don't enqueue Delete Module if opening campaign because it\nwill already have been deleted and new config loaded and we create\na race condition." shown="True" w415 {
          tunnel: w411 -> [_ w441]
          tunnel: w414 -> [_ w439]
          frame False {
          }
          frame True {
            n159 = Unbundle By Name(w441) -> ("PRM Config.GUID"=w440:string)
            n160 = call-poly "Enqueue Message.vi"("Message Data"=w440, "Message"="Delete Module", "Message Queue"=w439) -> ()  [unwired: 7 in, 2 out]
          }
        }
        n161 = Merge Errors(w408, w423) -> (w405:errorcluster)
        n162 = Unbundle By Name(w411) -> ("PRM Config.Process Name"=w406:string)
        n163 = call "Generate Temporary Report.vi"("error in (no error)"=w405, "Line of Events"=string[] ["Exited"], "Module Name"=w406) -> ("error out"=w404:errorcluster)  [unwired: 8 in]
        n164 = Concatenate Strings(w406, " Exit" ("text")) -> (w412:string)
        n165 = call "Write to Log File.vi"("error in"=w404, "text"=w412) -> ()  [unwired: 9 in, 1 out]
      }
      frame "Init UI Refs" {
        # "Enable: Start, Exit, Settings\nDisable: Stop"
        # "Init UI Refs - Store control references for UI controls.  Also enable/disable controls appropriately."
        n166 = property class="VI"("Front Panel.Closeable"=TRUE ("Front Panel Window:Closeable")) -> ()  [unwired: 2 in, 2 out]
        n167 = control-ref of="Status"() -> (w448:refnum<vi>)
        n168 = control-ref of="Exit"() -> (w445:refnum<vi>)
        n169 = Bundle By Name(cluster=w451, "Status Ref"=w448, "Exit Ref"=w445) -> (w450:T8)
        n170 = Build Array(w445) -> (w447:refnum<vi>[])
        n171 = call "Set Enable State on Multiple Controls.vi"("Enable?"=TRUE, "Controls"=w447) -> ()  [unwired: 10 in]
      }
      frame "Initialize" {
        # "Initialize - Get configuration settings, then message the UI to initialize, and broadcast the settings to the other message loops."
        n172 = property class="VI" props=["FP.State"]() -> (reference out=w459:refnum<vi>)  [unwired: 2 in, 2 out]
        n173 = call-poly "Enqueue Message.vi"("error in (no error)"=w462, "Message"="Init UI Refs", "Message Queue"=w467) -> ("error out"=w465:errorcluster, "dup Message Queue"=w466:refnum<queue>)  [unwired: 7 in]
        n174 = call-poly "Enqueue Message.vi"("error in (no error)"=w465, "Message"="Broadcast Settings", "Message Queue"=w466) -> ("error out"=w473:errorcluster, "dup Message Queue"=w472:refnum<queue>)  [unwired: 7 in]
        n175 = call "Make Child and Move.vi"("Process Name"=w458, "Name of Parent Panel"=w461, "New Center Coords"=w460, "VI in"=w459) -> ()  [unwired: 8 in]
        n176 = call-poly "Enqueue Message.vi"("error in (no error)"=w473, "Message Data"="Ready..." ("Ready..."), "Message"="Update Status", "Message Queue"=w472) -> ("error out"=w454:errorcluster)  [unwired: 6 in, 1 out]
        n177 = Unbundle By Name(w453) -> ("PRM Config.Process Name"=w457:string)
        n178 = Concatenate Strings(w457, " Initialize" ("text")) -> (w455:string)
        n179 = call "Write to Log File.vi"("error in"=w454, "text"=w455) -> ()  [unwired: 9 in, 1 out]
      }
      frame "Sequence Update" {
        # "Update the Sequence settings from the Sequence Dialog"
        # "Launch the Settings Dialog when the user clicks the 'Settings' button."
        n180 = in-place {
          in-place-border: w482 -> [w492]
          n181 = in-place-cluster #1(w475) -> ("PRM Config"=w487:T3)
          n182 = Variant To Data(type=T17 {"Auto?"=TRUE, "Manual Entry"=0.0, "Setpoint"=0.0} ("Cluster"), Variant=w492) -> (data=w491:T17)  [unwired: 1 in, 1 out]
          n183 = Unbundle By Name(w491) -> ("Auto?"=w490:bool, "Manual Entry"=w489:dbl, "Setpoint"=w488:dbl)
          n184 = Bundle By Name(cluster=w487, "Settings.Auto?"=w490, "Settings.Manual Entry"=w489, "Settings.PID 2 Parameters.Setpoint"=w488) -> (w486:T3)
          n185 = in-place-cluster #1("PRM Config"=w486) -> (w474:T9)
        }
        n186 = call-poly "Enqueue Message.vi"("Message"="Broadcast Settings", "Message Queue"=w483) -> ("error out"=w481:errorcluster)  [unwired: 8 in, 1 out]
        n187 = Unbundle By Name(w474) -> ("PRM Config.Process Name"=w479:string)
        n188 = Merge Errors(w481) -> (w476:errorcluster)
        n189 = Concatenate Strings(w479, " Sequence Update" ("text")) -> (w477:string)
        n190 = call "Write to Log File.vi"("error in"=w476, "text"=w477) -> ()  [unwired: 9 in, 1 out]
      }
      frame "Logging Stopped" {
        # "Logic for determining what action to take when the logging has stopped."
        n191 = case shown="\"Waiting for Exit (Acq Stopped)\"" w502 {
          selector: w502 -> [w505 _ _ _ _]
          tunnel: [w505 UI_State."Waiting for Exit (Log Stopped)" ("UI State") UI_State."Waiting for Stop (Log Stopped)" ("UI State") UI_State."Idle" ("UI State") UI_State."Idle" ("UI State")] -> w501
          tunnel: w500 -> [w504 w506 w508 w514 w520]
          tunnel: [w504 w506 w508 w513 w519] -> w495
          tunnel: w499 -> [_ _ _ w512 w518]
          frame Default {
          }
          frame "Waiting for Exit", "Waiting for Exit (Log Stopped)" {
          }
          frame "Waiting for Stop", "Waiting for Stop (Log Stopped)" {
          }
          frame "Waiting for Exit (Acq Stopped)" {
            # "If we are waiting to exit, and the acquisition has already stopped, then the \"Logging Stopped\" message indicates that it is time to exit."
            n192 = call-poly "Enqueue Message.vi"("Priority Message? (F)"=TRUE, "error in (no error)"=w514, "Message"="Exit", "Message Queue"=w512) -> ("error out"=w513:errorcluster)  [unwired: 6 in, 1 out]
          }
          frame "Waiting for Stop (Acq Stopped)" {
            # "If we are waiting to stop, and the acquisition has already stopped, then the \"Logging Stopped\" message indicates that it is time to stop."
            n193 = call-poly "Enqueue Message.vi"("error in (no error)"=w520, "Message Data"="Ready..." ("Message"), "Message"="Update Status", "Message Queue"=w518) -> ("error out"=w519:errorcluster)  [unwired: 6 in, 1 out]
          }
        }
        n194 = Unbundle By Name(w494) -> ("PRM Config.Process Name"=w498:string)
        n195 = Concatenate Strings(w498, " Logging Stopped" ("text")) -> (w496:string)
        n196 = call "Write to Log File.vi"("error in"=w495, "text"=w496) -> ()  [unwired: 9 in, 1 out]
      }
      frame "Open Settings Dialog" {
        # "Duplicate this frame when creating new messages.  Change this comment in the duplicated frame to describe this message."
        n197 = in-place {
          # "Keep track of how many times \nthe window has been opened"
          n198 = in-place-cluster #2(w529) -> ("PRM Config.Settings Load Count"=w535:i32)
          n199 = Increment(x=w535) -> (x+1=w534:i32)
          n200 = in-place-cluster #2("PRM Config.Settings Load Count"=w534) -> (w527:T9)
        }
        n201 = call-by-ref "?"("error in (no error)"=w525, "UI State"=w528, "Message Queues"=w526, "PRM State Cluster In"=w527) -> ("error out"=w522:errorcluster, "Cancelled?"=w524:bool, "PRM State Cluster Out"=w523:T9)  [unwired: 6 in, 3 out]
        n202 = Unbundle By Name(w523) -> ("PRM Config.Settings.Input Channel Tag Name"=→"Input Channel":string)
        n203 = case shown="False" w524 {
          tunnel: w522 -> [w537 w540]
          tunnel: [w536 w540] -> w531
          tunnel: w532 -> [w539 _]
          frame False {
            n204 = call-poly "Enqueue Message.vi"("error in (no error)"=w537, "Message"="Broadcast Settings", "Message Queue"=w539) -> ("error out"=w536:errorcluster)  [unwired: 7 in, 1 out]
          }
          frame True {
          }
        }
      }
      frame "Start" {
        # "We only have one loop but i've kept this in anyway"
        # "Clear chart"
        # "Message Acquisition and Logging loops to start"
        # "Enable: Stop\nDisable: Start, Exit, Settings"
        # "Start - Enable/Disable buttons appropriately for an acquisition that has started, and update status display."
        n205 = Unbundle By Name(w564) -> ("Trigger Ref"=w555:refnum<vi>, "Stop Ref"=w556:refnum<vi>, "Start Ref"=w559:refnum<vi>, "Exit Ref"=w558:refnum<vi>, "Settings Ref"=w557:refnum<vi>, "Data Ref"=w547:refnum<vi>)
        n206 = disable-structure shown="Enabled" {
          disable-tunnel: [w568 w570] -> w551
          disable-tunnel: w550 -> [w567 w571]
          disable-tunnel: [w566 w571] -> w549
          disable-tunnel: w548 -> [w565 w570]
          frame Disabled {
            n207 = call-poly "Enqueue Message.vi"("error in (no error)"=w565, "Message"="Broadcast settings", "Message Queue"=w567) -> ("error out"=w568:errorcluster, "dup Message Queue"=w566:refnum<queue>)  [unwired: 7 in]
          }
          frame Enabled {
          }
        }
        n208 = property class="WFChart (strict)"(reference=w547, "History Data"=waveform(dbl)[][] []) -> ()  [unwired: 1 in, 2 out]
        n209 = Build Array(w559, w558, w557) -> (w562:refnum<vi>[])
        n210 = Build Array(w555, w556) -> (w561:refnum<vi>[])
        n211 = call "Set Enable State on Multiple Controls.vi"("Enable?"=TRUE, "Controls"=w561) -> ()  [unwired: 10 in]
        n212 = call "Set Enable State on Multiple Controls.vi"("Enable?"=FALSE, "Controls"=w562) -> ()  [unwired: 10 in]
        n213 = call-poly "Enqueue Message.vi"("error in (no error)"=w551, "Message"="Start Loops", "Message Queue"=w549) -> ("error out"=w552:errorcluster)  [unwired: 7 in, 1 out]
        n214 = Merge Errors(w552) -> (w541:errorcluster)
        n215 = Unbundle By Name(w543) -> ("PRM Config.Process Name"=w542:string)
        n216 = Concatenate Strings(w542, " Start" ("text")) -> (w544:string)
        n217 = call "Write to Log File.vi"("error in"=w541, "text"=w544) -> ()  [unwired: 9 in, 1 out]
      }
      frame "Start Loops" {
        # "I'm not entirly sure where we would have a second Process Name in a module but i'm leaving it for now"
        # "Message Acquisition and Logging loops to start"
        # "Start - Enable/Disable buttons appropriately for an acquisition that has started, and update status display."
        n218 = Build Array(w580) -> (w579:refnum<queue>[])
        n219 = Unbundle By Name(w578) -> ("PRM Config.Process Name"=w572:string)
        n220 = for {
          tunnel: w576 -> [w586]
          tunnel: [w585] -> w577 mode=indexing
          tunnel: w579 -> [w584] mode=indexing
          tunnel: w572 -> [w583]
          n221 = call-poly "Enqueue Message.vi"("error in (no error)"=w586, "Message Data"=w583, "Message"="Start", "Message Queue"=w584) -> ("error out"=w585:errorcluster)  [unwired: 6 in, 1 out]
        }
        n222 = Merge Errors(w576, w577) -> (w574:errorcluster)
        n223 = call "Generate Temporary Report.vi"("error in (no error)"=w574, "Line of Events"=string[] ["Started"], "Module Name"=w572) -> ("error out"=w573:errorcluster)  [unwired: 8 in]
      }
      frame "Start Log" {
        # "I'm not entirly sure where we would have a second Process Name in a module but i'm leaving it for now"
        # "Message Acquisition and Logging loops to start"
        # "Start - Enable/Disable buttons appropriately for an acquisition that has started, and update status display."
        n224 = Build Array(w593) -> (w592:refnum<queue>[])
        n225 = Unbundle By Name(w590) -> ("PRM Config.Process Name"=w591:string)
        n226 = for {
          tunnel: w588 -> [w600]
          tunnel: [w599] -> w589 mode=indexing
          tunnel: w592 -> [w598] mode=indexing
          tunnel: w591 -> [w597]
          n227 = call-poly "Enqueue Message.vi"("error in (no error)"=w600, "Message Data"=w597, "Message"="Start Log", "Message Queue"=w598) -> ("error out"=w599:errorcluster)  [unwired: 6 in, 1 out]
        }
        n228 = property class="VI"("Front Panel.Title"=w591) -> ()  [unwired: 2 in, 2 out]
        n229 = Merge Errors(w588, w589) -> (w596:errorcluster)
      }
      frame "Stop" {
        # "Stop Pauses the engine"
        # "Enable: Start, Exit, Settings\nDisable: Stop"
        # "Stop - Enable/Disable buttons appropriately for an acquisition that has stopped, and update status display."
        n230 = Unbundle By Name(w623) -> ("Trigger Ref"=w614:refnum<vi>, "Stop Ref"=w615:refnum<vi>, "Start Ref"=w618:refnum<vi>, "Exit Ref"=w617:refnum<vi>, "Settings Ref"=w616:refnum<vi>)
        n231 = call-poly "Enqueue Message.vi"("error in (no error)"=w611, "Message Data"="Ready..." ("Ready..."), "Message"="Update Status", "Message Queue"=w626) -> ("error out"=w609:errorcluster)  [unwired: 6 in, 1 out]
        n232 = Build Array(w618, w617, w616) -> (w621:refnum<vi>[])
        n233 = Build Array(w614, w615) -> (w620:refnum<vi>[])
        n234 = call-poly "Enqueue Message.vi"("error in (no error)"=w609, "Message"="Pause", "Message Queue"=w610) -> ("error out"=w607:errorcluster)  [unwired: 7 in, 1 out]
        n235 = call "Set Enable State on Multiple Controls.vi"("Enable?"=FALSE, "Controls"=w620) -> ()  [unwired: 10 in]
        n236 = call "Set Enable State on Multiple Controls.vi"("Enable?"=TRUE, "Controls"=w621) -> ()  [unwired: 10 in]
        n237 = case shown="\"Waiting for Exit\"" w612 {
          selector: w612 -> [_ w628]
          tunnel: [UI_State."Waiting for Stop" ("UI State") w628] -> w613
          frame Default {
          }
          frame "Waiting for Exit" {
          }
        }
        n238 = Merge Errors(w607) -> (w605:errorcluster)
        n239 = Unbundle By Name(w603) -> ("PRM Config.Process Name"=w602:string)
        n240 = call "Generate Temporary Report.vi"("error in (no error)"=w605, "Line of Events"=string[] ["Stopped"], "Module Name"=w602) -> ("error out"=w604:errorcluster)  [unwired: 8 in]
      }
      frame "Update Status" {
        # "Update Display - Convert the message data to a string to display in the Status indicator."
        n241 = Unbundle By Name(w635) -> ("Trigger Ref"=w631:refnum<vi>, "Stop Ref"=w634:refnum<vi>)
        n242 = Variant To Data(error in=w639, type="", Variant=w638) -> (data=w632:string, error out=w636:errorcluster)
        "Status" <- w632
        n243 = property class="Bool"(reference=w634) -> ("DisabledEnum"=w633:T18)  [unwired: 1 in, 2 out]
        n244 = case shown="\"Enabled\"" w633 {
          tunnel: w632 -> [w643 _]
          tunnel: w631 -> [w644 _]
          frame "Enabled" {
            # "Disable the Force Trigger only while we are logging."
            n245 = Build Array(w644) -> (w645:refnum<vi>[])
            n246 = Not Equal?(x="Logging" ("Logging"), y=w643) -> (x != y?=w641:bool)
            n247 = call "Set Enable State on Multiple Controls.vi"("Enable?"=w641, "Controls"=w645) -> ()  [unwired: 10 in]
          }
          frame "Disabled", Default {
          }
        }
        n248 = Merge Errors(w636) -> (w640:errorcluster)
      }
      frame Default {
        # "'Default' case only runs if there is a message that isn't defined in any of the other cases.  Output a programming error."
        n249 = Concatenate Strings("The invalid message string " ("string"), w651, " was received in 4-20mA Main" ("string")) -> (w647:string)
        n250 = Bundle By Name(cluster=errorcluster {"status"=TRUE, "code"=1, "source"=""} ("error constant"), "source"=w647) -> (w646:errorcluster)
      }
    }
    n251 = call "Error Handler - Message Handling Loop.vi"("error in (no error)"=w181, "Message Queue"=w165) -> ("dup error in"=w180:errorcluster)  [unwired: 8 in, 1 out]
  }
  n252 = call "Main Loop.vi"("error in (no error)"=w9, "Chart Notifier"=w17, "Message Queues"=w18) -> ("error out"=w19:errorcluster)  [unwired: 8 in]
  n253 = Release Queue(queue=w6) -> ()  [unwired: 2 in, 3 out]
  n254 = Unregister For Events(event registration refnum=w25, error in=w30) -> (error out=w26:errorcluster)
  n255 = Close Reference(reference=w16) -> ()  [unwired: 1 in, 1 out]
  n256 = Release Queue(queue=w5) -> ()  [unwired: 2 in, 3 out]
  n257 = Release Queue(queue=w3) -> ()  [unwired: 2 in, 3 out]
  n258 = Merge Errors(w26, w31, w9, w19) -> (w29:errorcluster)
  n259 = call "Destroy User Event - Stop.vi"("error in (no error)"=w29, "User Event - Stop"=w27) -> ("error out"=w11:errorcluster)  [unwired: 9 in]
  n260 = flat-sequence {
    tunnel: w11 -> [_]
    frame #0 {
      n261 = invoke class="VI" method="FP.Close"() -> ()  [unwired: 3 in, 3 out]
    }
  }
